vi "Get Number Of Unhandled Errors.vi"(3 "Errors in current one-second interval":T2[](array[typedef])) -> (0 "At least one unhandled error?":bool, 1 "Unhandled Errors":T1[](array[typedef]))   [LabVIEW 2016, in "Error Manager.lvlib"]
doc: "Blank VI with error handling."
uses:
  Error Manager.lvlib
  Unhandled Error (cluster).ctl
  Error in current one-second interval (cluster).ctl
panel:
  # "Input\nInputs to the VI"
  # "Development\nControls or indicators that are useful for development or testing, but which are not outputs of the VI."
  # "Output\nOutputs of the VI"
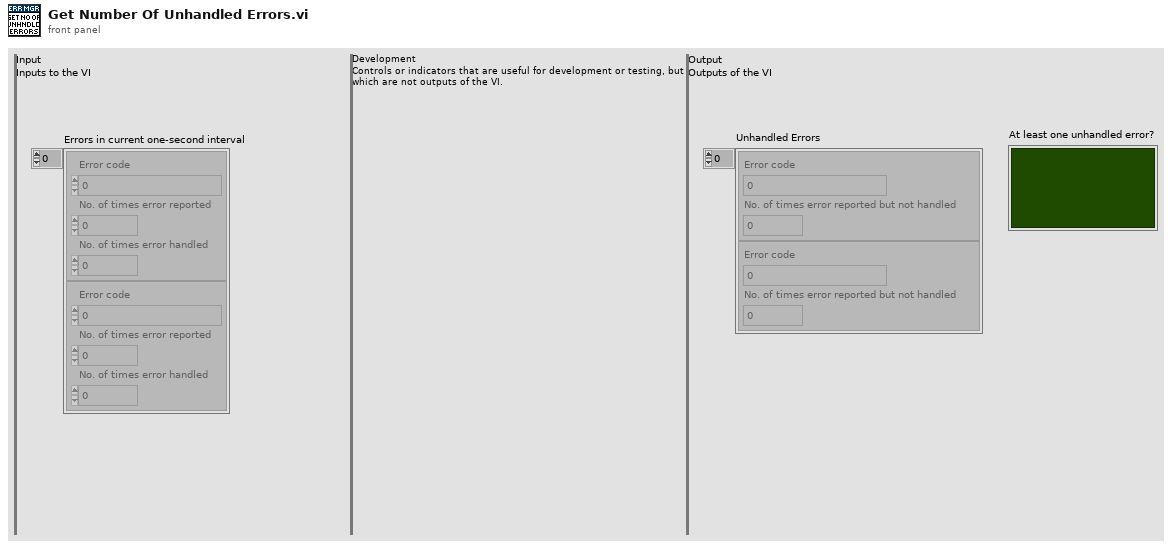
[diagram p1: front panel]
types:
  T1 = typedef "Error Manager.lvlib/Unhandled Error (cluster).ctl" = cluster{"Error code":i32, "No. of times error reported but not handled":u32}
  T2 = typedef "Error Manager.lvlib/Error in current one-second interval (cluster).ctl" = cluster{"Error code":i32, "No. of times error reported":u32, "No. of times error handled":u32}
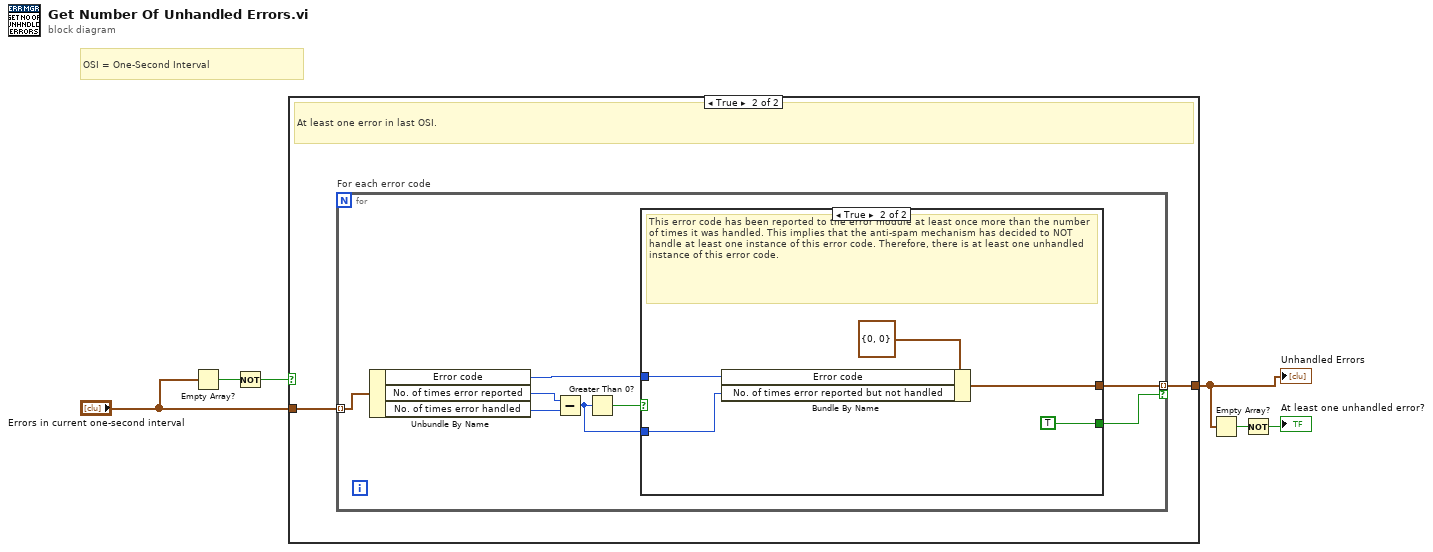
[diagram p0: block diagram]
diagram:
  # "OSI = One-Second Interval"
  n1 = Empty Array?(array="Errors in current one-second interval") -> (empty?=w5:bool)
  n2 = Not(x=w5) -> (.not. x?=w4:bool)
  n3 = case shown="True" w4 {
    tunnel: "Errors in current one-second interval" -> [_ w8]
    tunnel: [_ w7] -> w3
    frame False {
      # "No errors in last OSI. This implies no Unhandled Errors. That's ok."
    }
    frame True {
      # "At least one error in last OSI."
      n4 = for "For each error code" {
        tunnel: w8 -> [w16] mode=indexing
        tunnel: [w10] -> w7 mode=indexing if=w9
        n5 = Unbundle By Name(w16) -> ("Error code"=w13:i32, "No. of times error reported"=w15:u32, "No. of times error handled"=w14:u32)
        n6 = Subtract(x=w15, y=w14) -> (x-y=w11:u32)
        n7 = Greater Than 0?(x=w11) -> (x > 0?=w12:bool)
        n8 = case shown="True" w12 {
          tunnel: w13 -> [_ w20]
          tunnel: w11 -> [_ w19]
          tunnel: [_ w18] -> w10
          tunnel: [_ TRUE] -> w9
          frame False {
            # "All instances of this error code have been handled. There are no unhandled instances of this error code."
          }
          frame True {
            # "This error code has been reported to the error module at least once more than the number of times it was handled. This implies that the anti-spam mechanism has decided to NOT handle at least one instance of this error code. Therefore, there is at least one unhandled instance of this error code."
            n9 = Bundle By Name(cluster=T1 {"Error code"=0, "No. of times error reported but not handled"=0} ("Unhandled Error"), "Error code"=w20, "No. of times error reported but not handled"=w19) -> (w18:T1)
          }
        }
      }
    }
  }
  "Unhandled Errors" <- w3
  n10 = Empty Array?(array=w3) -> (empty?=w2:bool)
  n11 = Not(x=w2) -> (.not. x?=→"At least one unhandled error?":bool)
